vi "Initialize Instrument.vi"(8 "error in (no error)":errorcluster, 10 "Reset":bool, 11 "Manual PSU in":refnum<class "Manual PSU.lvclass">) -> (0 "error out":errorcluster, 3 "Manual PSU out":refnum<class "Manual PSU.lvclass">)   [LabVIEW 2020, in "Manual PSU.lvclass"]
uses:
  Manual PSU.lvclass
  C:/Sandbox/Git_Sandbox/WiSpry Test Framework source code (LV20)/WiSpry Test Framework/Instruments/Instrument.lvclass
  Instrument.lvclass/Instrument.ctl
  Instrument.lvclass
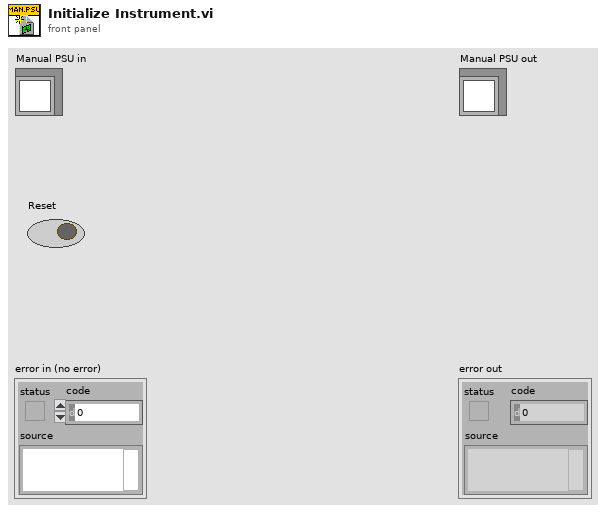
[diagram p1: front panel]
types:
  T1 = typedef "Instrument.lvclass/Interface String Cluster.ctl" = cluster{"Interface":string, "IDN string":string, "Instance":i32}
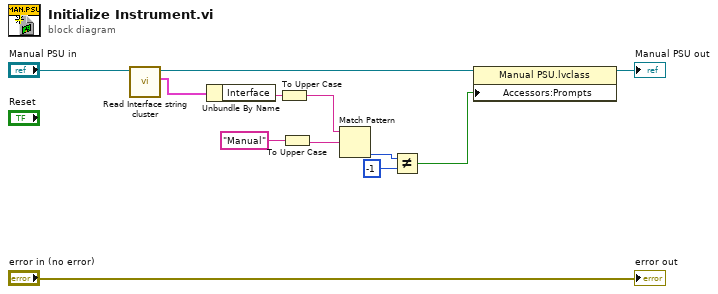
[diagram p0: block diagram]
diagram:
  n1 = call "Read Interface string cluster.vi"("Instrument in"="Manual PSU in") -> ("Interface sting cluster"=w10:T1, "Instrument out"=w9:refnum<class "Manual PSU.lvclass">)  [unwired: 9 in]
  n2 = Unbundle By Name(w10) -> ("Interface"=w6:string)
  n3 = To Upper Case(1:w6) -> (0:w7:string)
  n4 = To Upper Case(1:"Manual" ("string")) -> (0:w5:string)
  n5 = Match Pattern(string=w7, regular expression=w5) -> (offset past match=w3:i32)  [unwired: 1 in, 3 out]
  n6 = Not Equal?(x=w3, y=-1) -> (x != y?=w1:bool)
  n7 = property class="Manual PSU.lvclass"(reference=w9, "Accessors:Prompts"=w1) -> (reference out=→"Manual PSU out":refnum<class "Manual PSU.lvclass">)  [unwired: 1 in, 1 out]
  "error out" <- "error in (no error)"
